vi "draw_map.vi"(3 "error in":errorcluster, 4 "Message":string="{\t\t\"gis_anchor\": {\n\t\t\t\"x\": 40.410262,\n\t\t\t\"y\": -79.948172,\n\t\t\t\"z\": 1\n\t\t},\n\t\t\"orientation\": -16.5,\n\t\t\"point_delta\": 100.0,\n\t\t\"coordinates\": \"world\",\n   \"format\": \"point_array\"\n}\n", 5 "Vehicle Start Position":i32=1 min=-1 max=2 step=1, 6 "simx in":T1) -> (0 "error out":errorcluster, 2 "simx out":T1={"Config"={"Trajectory"={"Number of frames"=0, "Frame number"=0, "Trajectory"=""}, "Weather"={"id"=""}}, "Connections"={"Simulator Connection"=refnum, "server_ip"="127.0.0.1", "Port"=0, "Sensor connections"=[]}, "Map"={"lanes"={"x"=[], "y"=[], "z"=[]}, "StartPosition"={"start_points"={"locations"=[], "rotations"=[], "type"=[]}, "StartRotation"=[], "StartLocation"=[]}, "Draw Map Size"={"Width"=0, "Height"=0}, "DrawArea"={"min_Y"=0.0, "min_X"=0.0, "Scale X"=0.0, "Scale Y"=0.0}, "Map"=bytes[0], "Map Geojson"=""}})   [LabVIEW 2025]
doc: "Query the start points from the map."
uses:
  controls/simx_connection.ctl
  controls/config.ctl
  controls/trajectory.ctl
  controls/weather.ctl
  controls/connections.ctl
  controls/start_points.ctl
  <vilib>/Utility/miscctls.llb/LVBoundsTypeDef.ctl
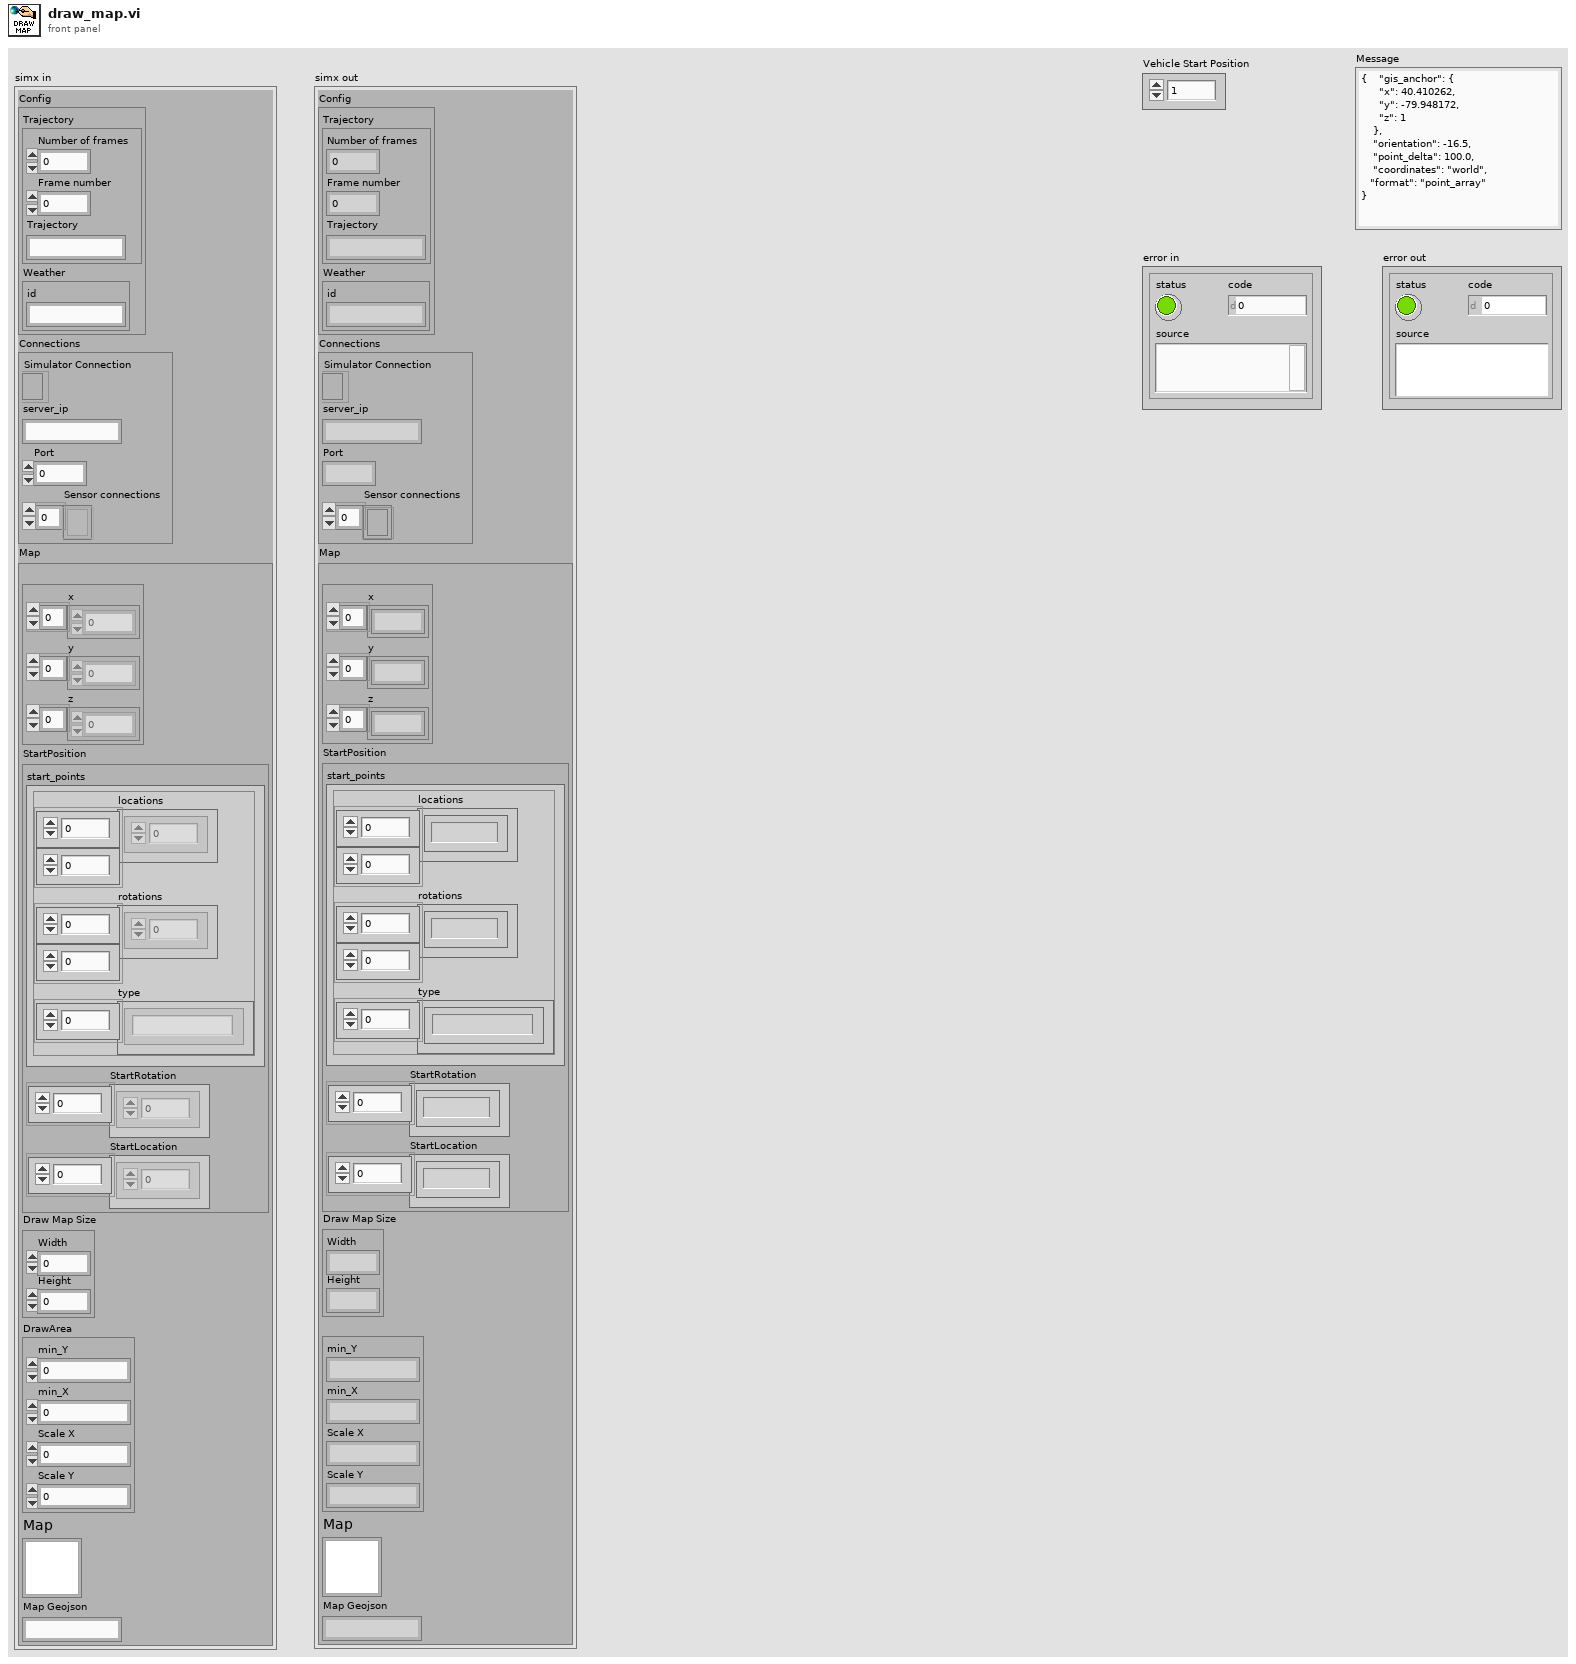
[diagram p1: front panel]
types:
  T1 = typedef "simx_connection.ctl" = cluster{"Config":T2, "Connections":T5, "Map":cluster{"lanes":cluster{"x":dbl[], "y":dbl[], "z":dbl[]}, "StartPosition":cluster{"start_points":T6, "StartRotation":dbl[], "StartLocation":dbl[]}, "Draw Map Size":T7, "DrawArea":cluster{"min_Y":dbl, "min_X":dbl, "Scale X":dbl, "Scale Y":dbl}, "Map":picture, "Map Geojson":string}}
  T2 = typedef "config.ctl" = cluster{"Trajectory":T3, "Weather":T4}
  T3 = typedef "trajectory.ctl" = cluster{"Number of frames":i32, "Frame number":i32, "Trajectory":string}
  T4 = typedef "weather.ctl" = cluster{"id":string}
  T5 = typedef "connections.ctl" = cluster{"Simulator Connection":refnum<k5>, "server_ip":string, "Port":i32, "Sensor connections":refnum<k5>[]}
  T6 = typedef "start_points.ctl" = cluster{"locations":dbl[][], "rotations":dbl[][], "type":string[]}
  T7 = typedef "LVBoundsTypeDef.ctl" = cluster{"Width":u32, "Height":u32}
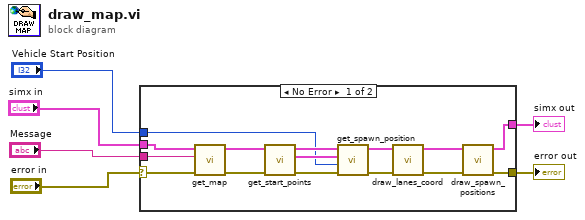
[diagram p0: block diagram]
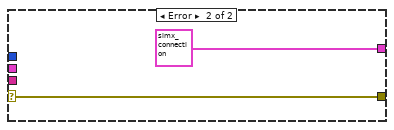
[diagram p2: hidden frame]
diagram:
  n1 = case shown="No Error" "error in" {
    selector: "error in" -> [w19 w22]
    tunnel: "simx in" -> [w20 _]
    tunnel: [w15 T1 {"Config"={"Trajectory"={"Number of frames"=0, "Frame number"=0, "Trajectory"=""}, "Weather"={"id"=""}}, "Connections"={"Simulator Connection"=refnum, "server_ip"="127.0.0.1", "Port"=0, "Sensor connections"=[]}, "Map"={"lanes"={"x"=[], "y"=[], "z"=[]}, "StartPosition"={"start_points"={"locations"=[], "rotations"=[], "type"=[]}, "StartRotation"=[], "StartLocation"=[]}, "Draw Map Size"={"Width"=0, "Height"=0}, "DrawArea"={"min_Y"=0.0, "min_X"=0.0, "Scale X"=0.0, "Scale Y"=0.0}, "Map"=bytes[0], "Map Geojson"=""}} ("monoDrive out")] -> w4
    tunnel: [w18 w22] -> w3
    tunnel: "Vehicle Start Position" -> [w7 _]
    tunnel: "Message" -> [w14 _]
    frame No Error {
      n2 = call "get_map.vi"("error in"=w19, "message"=w14, "simx in"=w20) -> ("error out"=w21:errorcluster, "simx out"=w13:T1)  [unwired: 3 in]
      n3 = call "get_start_points.vi"("error in"=w21, "simx in"=w13) -> ("error out"=w12:errorcluster, "Starting Points"=w8:T6, "simx out"=w11:T1)  [unwired: 3 in]
      n4 = call "get_spawn_position.vi"("error in"=w12, "Vehicle Start Position"=w7, "Starting Points"=w8, "simx in"=w11) -> ("error out"=w9:errorcluster, "simx out"=w10:T1)  [unwired: 2 in]
      n5 = call "draw_lanes_coord.vi"("error in"=w9, "monoDrive in"=w10) -> ("error out"=w16:errorcluster, "monoDrive out"=w17:T1)  [unwired: 4 in]
      n6 = call "draw_spawn_positions.vi"("error in"=w16, "simx in"=w17) -> ("error out"=w18:errorcluster, "simx out"=w15:T1)  [unwired: 4 in]
    }
    frame Error {
    }
  }
  "simx out" <- w4
  "error out" <- w3
